vi "Get Module Config.vi"(8 "error in (no error)":errorcluster, 11 "9235 in":refnum<class "9235.lvclass">) -> (0 "error out":errorcluster, 2 "Config Channels":dbl[](array[numeric]), 3 "9235 out":refnum<class "9235.lvclass">)   [LabVIEW 2019, in "Modules.lvlib" / "9235.lvclass"]
uses:
  9235.lvclass
  9235.lvclass/9235.ctl
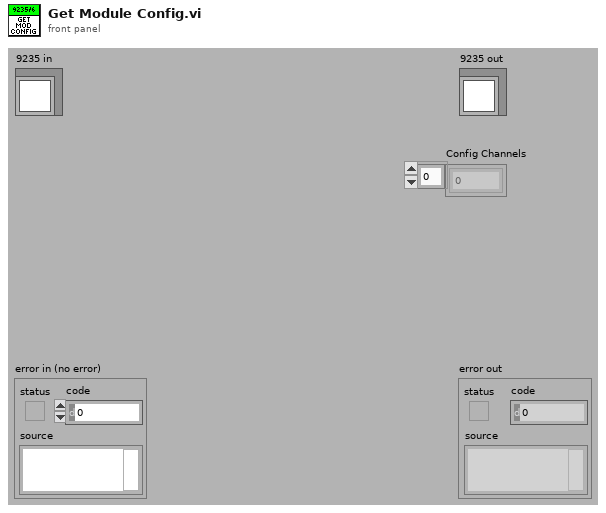
[diagram p1: front panel]
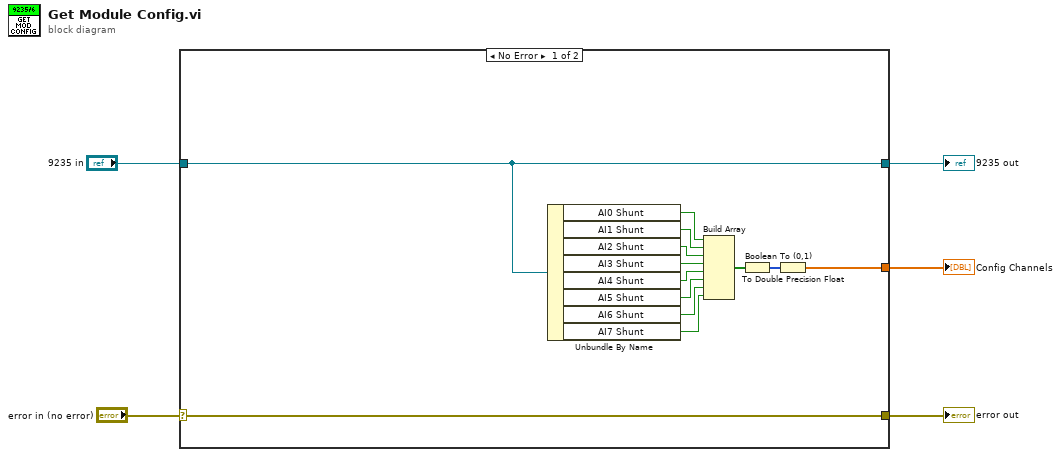
[diagram p0: block diagram]
diagram:
  n1 = case shown="No Error" "error in (no error)" {
    selector: "error in (no error)" -> [w18 w20]
    tunnel: "9235 in" -> [w17 w19]
    tunnel: [w18 w20] -> w3
    tunnel: [w17 w19] -> w2
    tunnel: [w10 _] -> w1
    frame No Error {
      n2 = Unbundle By Name(w17) -> ("AI0 Shunt"=w16:bool, "AI1 Shunt"=w15:bool, "AI2 Shunt"=w14:bool, "AI3 Shunt"=w13:bool, "AI4 Shunt"=w9:bool, "AI5 Shunt"=w8:bool, "AI6 Shunt"=w7:bool, "AI7 Shunt"=w6:bool)
      n3 = Build Array(w16, w15, w14, w13, w9, w8, w7, w6) -> (w12:bool[])
      n4 = Boolean To (0,1)(Boolean=w12) -> (0, 1=w11:i16[])
      n5 = To Double Precision Float(number=w11) -> (double precision float=w10:dbl[])
    }
    frame Error {
    }
  }
  "error out" <- w3
  "9235 out" <- w2
  "Config Channels" <- w1
